vi "emi_ Set Main Background.vi"(5 "VI Refnum(This vi)":refnum<vi>, 9 "error in (no error)":errorcluster) -> (6 "VI Refnum":refnum<vi>, 10 "error out":errorcluster)   [LabVIEW 2011]
doc: "Sets teh colors of teh Panel background to teh Main window system 01 color settings\nIf no VI ref in, then the VI containing this VI is used.\nIf VI has multiple panes, only the first pane will be used.\n\nOn error in: Does not run."
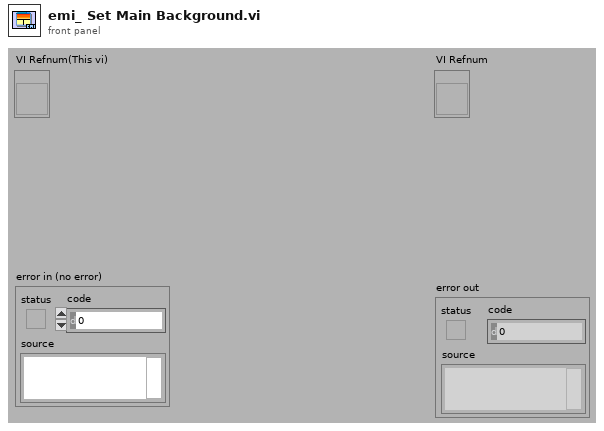
[diagram p1: front panel]
types:
  T1 = typedef "emi_System Colors.ctl" = cluster{"Main Top Panels":T2, "Main Botom Panels":T2, "Graphs":T2, "Dialogs":T2}
  T2 = typedef "_emi_ Color defenition.ctl" = cluster{"Type":T3, "Dark/Primary Color":u32, "Light/Secondary Color":u32, "Extra Color":u32}
  T3 = typedef "emi_List Of Graphix.ctl" = enum16{"FlatColor", "SharpGrad", "ShallowGrad", "GlasGradBord", "GlasGrad", "GlasGradBord 2"}
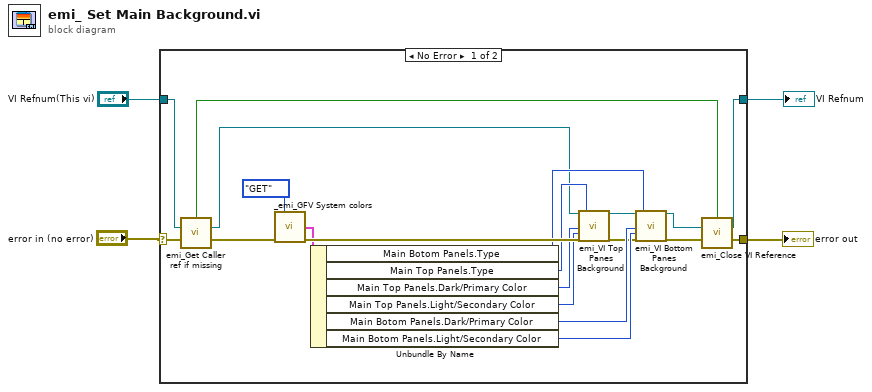
[diagram p0: block diagram]
diagram:
  n1 = case shown="No Error" "error in (no error)" {
    selector: "error in (no error)" -> [w23 w26]
    tunnel: [w21 w26] -> w4
    tunnel: "VI Refnum(This vi)" -> [w22 w25]
    tunnel: [w20 w25] -> w2
    frame No Error {
      n2 = call "emi_Get Caller ref if missing.vi"("VI Refnum(Calling VI)"=w22, "error in (no error)"=w23) -> ("Ref Generated"=w24:bool, "VI Refnum Out"=w7:refnum<vi>, "error out"=w8:errorcluster)  [unwired: 11 in]
      n3 = call "_emi_GFV System colors.vi"("Action(GET)"=enum16{"GET", "SET"}."GET", "error in (no error)"=w8) -> ("System background out"=w18:T1, "error out"=w19:errorcluster)  [unwired: 12 in]
      n4 = Unbundle By Name(w18) -> ("Main Botom Panels.Type"=w12:T3, "Main Top Panels.Type"=w13:T3, "Main Top Panels.Dark/Primary Color"=w14:u32, "Main Top Panels.Light/Secondary Color"=w15:u32, "Main Botom Panels.Dark/Primary Color"=w16:u32, "Main Botom Panels.Light/Secondary Color"=w17:u32)
      n5 = call "emi_VI Top Panes Background.vi"("VI Refnum(This VI)"=w7, "Dark(Black)"=w14, "Light(White)"=w15, "error in"=w19, "Graphic Type(Flat Color)"=w13) -> ("VI Refnum out"=w10:refnum<vi>, "error IO"=w9:errorcluster)  [unwired: 13 in]
      n6 = call "emi_VI Bottom Panes Background.vi"("VI Refnum(This VI)"=w10, "Dark(Black)"=w16, "Light(White)"=w17, "error in"=w9, "Graphic Type(Flat Color)"=w12) -> ("VI Refnum out"=w6:refnum<vi>, "error IO"=w5:errorcluster)  [unwired: 13 in]
      n7 = call "emi_Close VI Reference.vi"("Close ref?(T)"=w24, "VI Refnum"=w6, "error in (no error)"=w5) -> ("VI Refnum Out"=w20:refnum<vi>, "error out"=w21:errorcluster)  [unwired: 11 in]
    }
    frame Error {
    }
  }
  "error out" <- w4
  "VI Refnum" <- w2
